vi "metWeighted.vi"(0 "VSERTIM Path":string="C:\\Users\\Hesham\\Documents\\GitHub\\LabVIEW\\Wind Analysis\\C1\\tmseries\\node1") -> (1 "tmeanEx":dbl[][][](array[numeric]), 2 "tgemEx":dbl[][][](array[numeric]))   [LabVIEW 2018]
panel:
  out "array w/ subset deleted":dbl[][](array[numeric])
  out "gemEx":dbl[][][][](array[numeric])
  out "meanEx":dbl[][][][](array[numeric])
  # "is meanEX and genEX really necessary????"
  # "Season"
  # "Velocity Threshold"
  # "Probe Number"
  # "Angle"
  # "Season"
  # "Probe Number"
  # "Velocity Threshold"
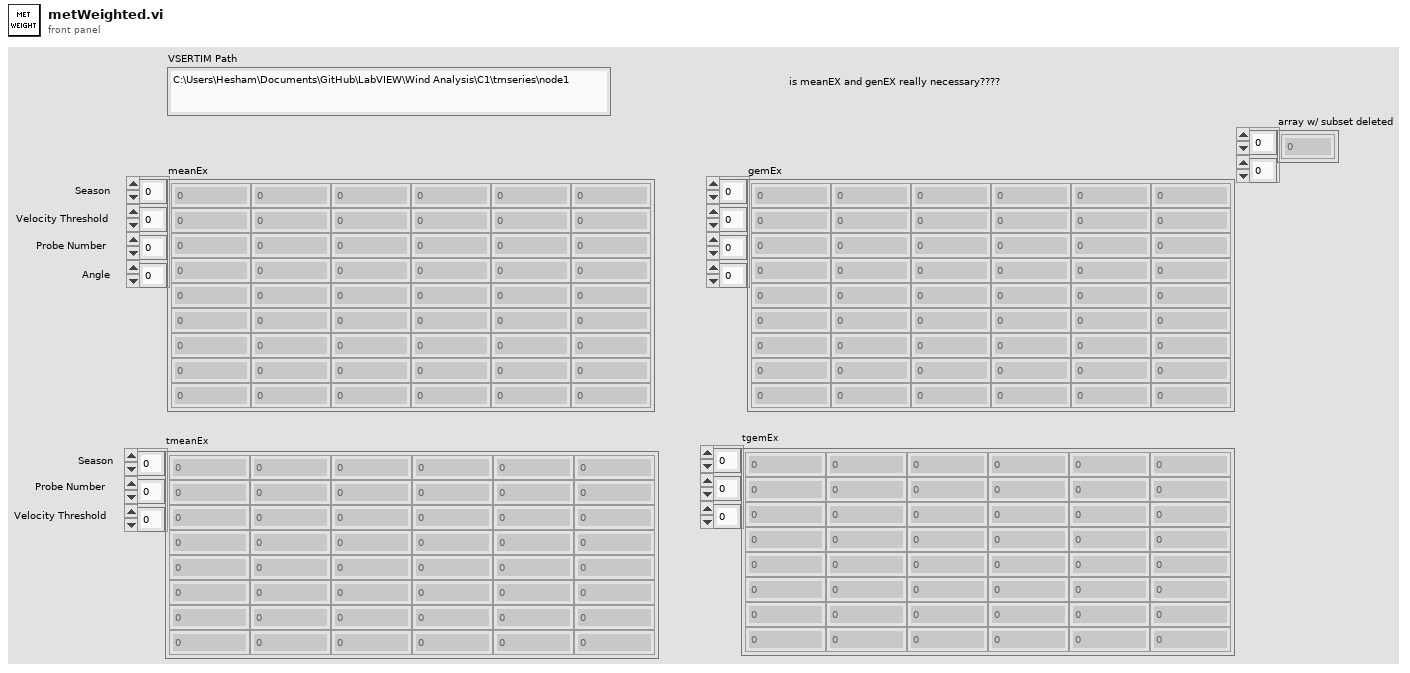
[diagram p1: front panel]
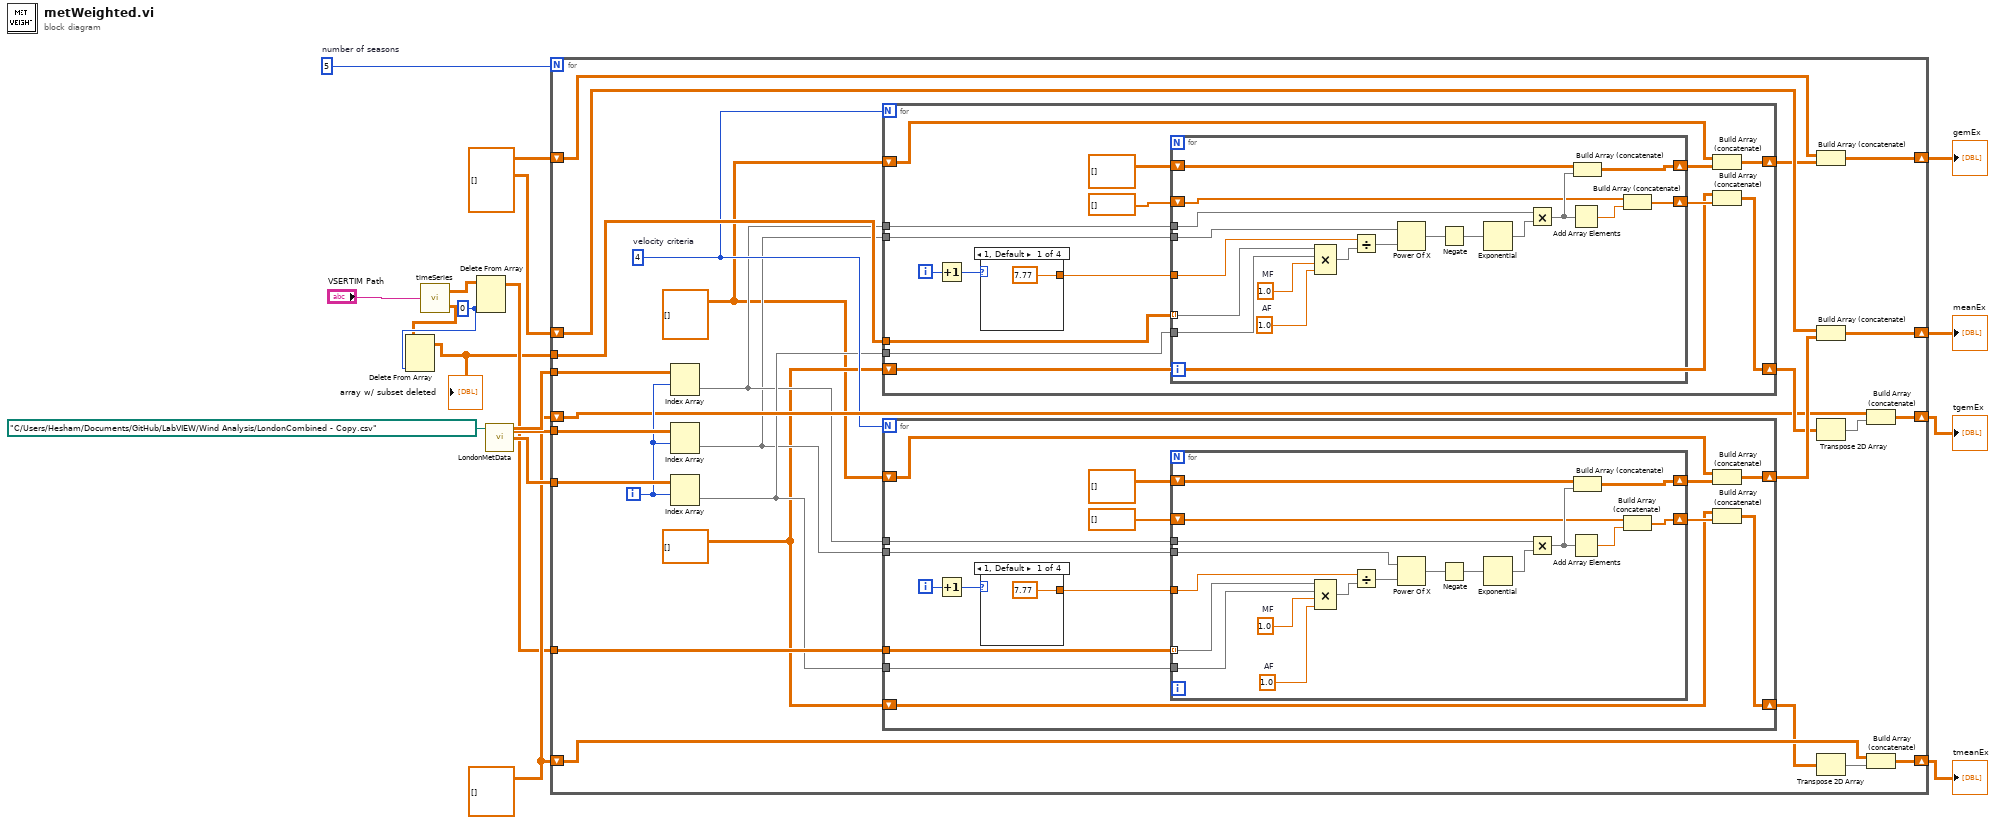
[diagram p0: block diagram]
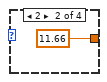
[diagram p2: hidden frame]
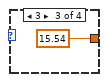
[diagram p3: hidden frame]
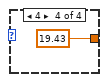
[diagram p4: hidden frame]
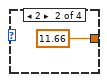
[diagram p5: hidden frame]
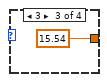
[diagram p6: hidden frame]
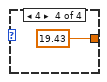
[diagram p7: hidden frame]
diagram:
  w3 = 0 ("disabled index (col)")
  w10 = dbl[][][] []
  w11 = dbl[][][][] []
  w17 = 5  # number of seasons
  n1 = call "timeSeries.vi"("Results Path"="VSERTIM Path") -> ("Mean VRs"=w5:dbl[][], "GEM VRs"=w2:dbl[][])
  n2 = Delete From Array(array=w2, index (col)=w3) -> (array with subset deleted=w1:dbl[][])  [unwired: 2 in, 1 out]
  "array w/ subset deleted" <- w1
  n3 = Delete From Array(array=w5, index (col)=w3) -> (array with subset deleted=w4:dbl[][])  [unwired: 2 in, 1 out]
  n4 = call "LondonMetData.vi"("Met Data File Path"=path "C:/Users/Hesham/Documents/GitHub/LabVIEW/Wind Analysis/LondonCombined - Copy.csv") -> ("k"=w13:dbl[][], "c"=w12:dbl[][], "p"=w14:dbl[][])  [unwired: 2 in]
  n5 = for {
    N: w17 -> [_]
    tunnel: w4 -> [w43]
    tunnel: w13 -> [w42]
    tunnel: w12 -> [w41]
    shift-right: [w39] -> w16
    shift-left: w11 -> [w38]
    shift-right: [w37] -> w15
    shift-left: w10 -> [w36]
    tunnel: w14 -> [w30]
    tunnel: w1 -> [w29]
    shift-right: [w26] -> w9
    shift-left: w11 -> [w27]
    shift-right: [w24] -> w8
    shift-left: w10 -> [w25]
    i -> [w28]
    w19 = dbl[][] []
    w18 = dbl[][][] []
    w23 = 4  # velocity criteria
    n6 = Index Array(array=w30, index (row)=w28) -> (element=w21:dbl[])  [unwired: 1 in]
    n7 = Index Array(array=w42, index (row)=w28) -> (element=w20:dbl[])  [unwired: 1 in]
    n8 = Index Array(array=w41, index (row)=w28) -> (element=w22:dbl[])  [unwired: 1 in]
    n9 = for {
      N: w23 -> [_]
      tunnel: w29 -> [w58]
      tunnel: w21 -> [w54]
      tunnel: w20 -> [w53]
      tunnel: w22 -> [w52]
      shift-right: [w50] -> w31
      shift-left: w18 -> [w49]
      shift-right: [w45] -> w32
      shift-left: w19 -> [w44]
      i -> [w57]
      n10 = Increment(x=w57) -> (x+1=w56:i32)
      n11 = case shown="1, Default" w56 {
        tunnel: [7.77 11.66 15.54 19.43] -> w55
        frame 1, Default {
        }
        frame 2 {
        }
        frame 3 {
        }
        frame 4 {
        }
      }
      n12 = for {
        tunnel: w54 -> [w75]
        tunnel: w53 -> [w69]
        tunnel: w52 -> [w65]
        tunnel: w58 -> [w71] mode=indexing
        shift-right: [w64] -> w51
        shift-left: dbl[][] [] -> [w74]
        tunnel: w55 -> [w67]
        shift-right: [w61] -> w46
        shift-left: dbl[] [] -> [w60]
        w72 = 1.0  # AF
        w66 = 1.0  # MF
        n13 = Compound Arithmetic op=MULTIPLY(w71, w65, w66, w72) -> (w59:dbl[])
        n14 = Divide(x=w67, y=w59) -> (x/y=w70:dbl[])
        n15 = Power Of X(1:w70, 2:w69) -> (0:w68:dbl[])
        n16 = Negate(x=w68) -> (-x=w73:dbl[])
        n17 = Exponential(1:w73) -> (0:w76:dbl[])
        n18 = Multiply(x=w75, y=w76) -> (x*y=w63:dbl[])
        n19 = Add Array Elements(numeric array=w63) -> (sum=w62:dbl)
        n20 = Build Array (concatenate)(w74, w63) -> (w64:dbl[][])
        n21 = Build Array (concatenate)(w60, w62) -> (w61:dbl[])
      }
      n22 = Build Array (concatenate)(w49, w51) -> (w50:dbl[][][])
      n23 = Build Array (concatenate)(w44, w46) -> (w45:dbl[][])
    }
    n24 = for {
      N: w23 -> [_]
      tunnel: w43 -> [w95]
      tunnel: w21 -> [w91]
      tunnel: w20 -> [w90]
      tunnel: w22 -> [w89]
      shift-right: [w87] -> w40
      shift-left: w18 -> [w86]
      shift-right: [w82] -> w35
      shift-left: w19 -> [w81]
      i -> [w94]
      n25 = Increment(x=w94) -> (x+1=w93:i32)
      n26 = case shown="1, Default" w93 {
        tunnel: [7.77 11.66 15.54 19.43] -> w92
        frame 1, Default {
        }
        frame 2 {
        }
        frame 3 {
        }
        frame 4 {
        }
      }
      n27 = for {
        tunnel: w91 -> [w112]
        tunnel: w90 -> [w105]
        tunnel: w89 -> [w101]
        tunnel: w95 -> [w108] mode=indexing
        shift-right: [w100] -> w88
        shift-left: dbl[][] [] -> [w111]
        tunnel: w92 -> [w103]
        shift-right: [w97] -> w83
        shift-left: dbl[] [] -> [w96]
        w109 = 1.0  # AF
        w102 = 1.0  # MF
        n28 = Compound Arithmetic op=MULTIPLY(w108, w101, w102, w109) -> (w107:dbl[])
        n29 = Divide(x=w103, y=w107) -> (x/y=w106:dbl[])
        n30 = Power Of X(1:w106, 2:w105) -> (0:w104:dbl[])
        n31 = Negate(x=w104) -> (-x=w110:dbl[])
        n32 = Exponential(1:w110) -> (0:w113:dbl[])
        n33 = Multiply(x=w112, y=w113) -> (x*y=w99:dbl[])
        n34 = Add Array Elements(numeric array=w99) -> (sum=w98:dbl)
        n35 = Build Array (concatenate)(w111, w99) -> (w100:dbl[][])
        n36 = Build Array (concatenate)(w96, w98) -> (w97:dbl[])
      }
      n37 = Build Array (concatenate)(w86, w88) -> (w87:dbl[][][])
      n38 = Build Array (concatenate)(w81, w83) -> (w82:dbl[][])
    }
    n39 = Build Array (concatenate)(w27, w31) -> (w26:dbl[][][][])
    n40 = Build Array (concatenate)(w38, w40) -> (w39:dbl[][][][])
    n41 = Transpose 2D Array(2D array=w32) -> (transposed array=w33:dbl[][])
    n42 = Transpose 2D Array(2D array=w35) -> (transposed array=w34:dbl[][])
    n43 = Build Array (concatenate)(w25, w33) -> (w24:dbl[][][])
    n44 = Build Array (concatenate)(w36, w34) -> (w37:dbl[][][])
  }
  "meanEx" <- w16
  "tmeanEx" <- w15
  "gemEx" <- w9
  "tgemEx" <- w8
